vi "Autonomous State Machine Tote.vi"   [LabVIEW 2014]
doc: "This VI is called when autonomous begins, and will automatically be terminated when autonomous ends. You can carry out timed or sensor driven robot movement independently without needing to return to the caller."
uses:
  <vilib>/Rock Robotics/WPI/RobotDrive/WPI_RobotDriveGetSetRefNum.vi
panel:
  # "Be sure to right-click and choose Data Operations>>Make Current Value default if you want to save the array values with the VI"
types:
  T1 = typedef "WPI_MotorControlDeviceRef.ctl" = cluster{"DeviceStatus":errorcluster, "Type":T2, "PWM":cluster{"Controller":T3, "PWM Channel":T4, "DeadBand":T5}, "CAN":cluster{"Device Number":u8, "Control Mode":T6, "Semaphore":T7, "Max Vout":dbl, "TalonSRX Control Mode":T8}, "Invert":bool, "TransformRef":T9, "InvTransformRef":T9}
  T2 = typedef "WPI_MotorControlType.ctl" = enum16{"PWM", "CAN", "CANTalonSRX"}
  T3 = typedef "FPGA_TypedefDigitalModule.ctl" = enum16{"Controller 1"}
  T4 = typedef "FPGA_DIOPWMChannel.ctl" = enum8{"PWM 0", "PWM 1", "PWM 2", "PWM 3", "PWM 4", "PWM 5", "PWM 6", "PWM 7", "PWM 8", "PWM 9", "PWM MXP 0", "PWM MXP 1", "PWM MXP 2", "PWM MXP 3", "PWM MXP 4", "PWM MXP 5", "PWM MXP 6", "PWM MXP 7", "PWM MXP 8", "PWM MXP 9", "Invalid"}
  T5 = typedef "WPI_PWMDeadband.ctl" = cluster{"Name":string, "maxPositivePwm":i32, "minPositivePwm":i32, "centerPwm":i32, "maxNegativePwm":i32, "minNegativePwm":i32, "angularRange":u16}
  T6 = typedef "WPI_CANJaguar_ControlMode.ctl" = enum8{"Percent VBus", "Current", "Speed", "Position", "Voltage"}
  T7 = typedef "Semaphore RefNum" = refnum<k1>
  T8 = typedef "WPI_CANTalonSRX_APIControlMode.ctl" = enum8{"Percent VBus", "Speed", "Position", "Slave", "Unchanged / Invalid"}
  T9 = typedef "WPI_PWMTransform_ConPane.ctl" = refnum<vi>
  T10 = typedef "WPI_RobotDriveDevRef.ctl" = cluster{"DevStatus":errorcluster, "Motors[]":T1[], "Square Inputs":bool, "Max Output":dbl}
  T11 = typedef "WPI_SwitchDevRef.ctl" = cluster{"DevStatus":errorcluster, "DIO Channel":T12, "Controller":T3, "CntIndex":T13, "Normally Closed":bool}
  T12 = typedef "FPGA_DIOChannel.ctl" = enum8{"DIO 0", "DIO 1", "DIO 2", "DIO 3", "DIO 4", "DIO 5", "DIO 6", "DIO 7", "DIO 8", "DIO 9", "DIO MXP 0", "DIO MXP 1", "DIO MXP 2", "DIO MXP 3", "DIO MXP 4", "DIO MXP 5", "DIO MXP 6", "DIO MXP 7", "DIO MXP 8", "DIO MXP 9", "DIO MXP 10", "DIO MXP 11", "DIO MXP 12", "DIO MXP 13", "DIO MXP 14", "DIO MXP 15", "Invalid"}
  T13 = typedef "FPGA_CounterCtrSystemIndex.ctl" = enum8{"Ctr 0", "Ctr 1", "Ctr 2", "Ctr 3", "Ctr 4", "Ctr 5", "Ctr 6", "Ctr 7", "Invalid"}
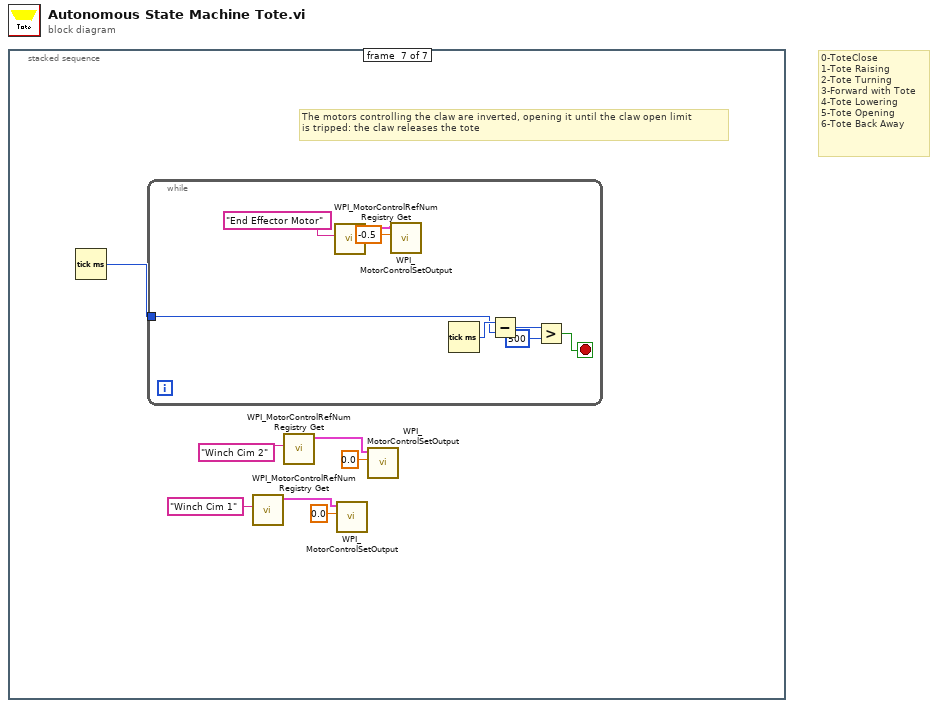
[diagram p0: block diagram]
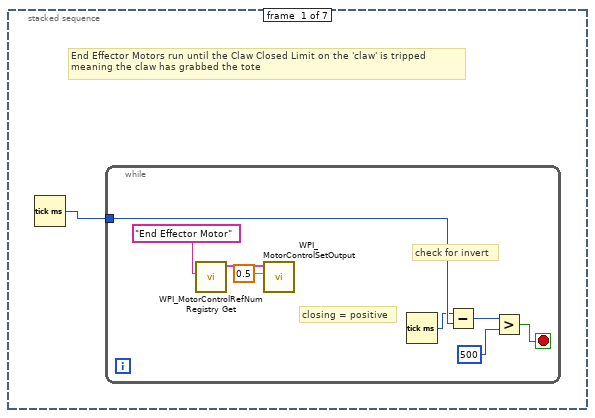
[diagram p2: hidden frame]
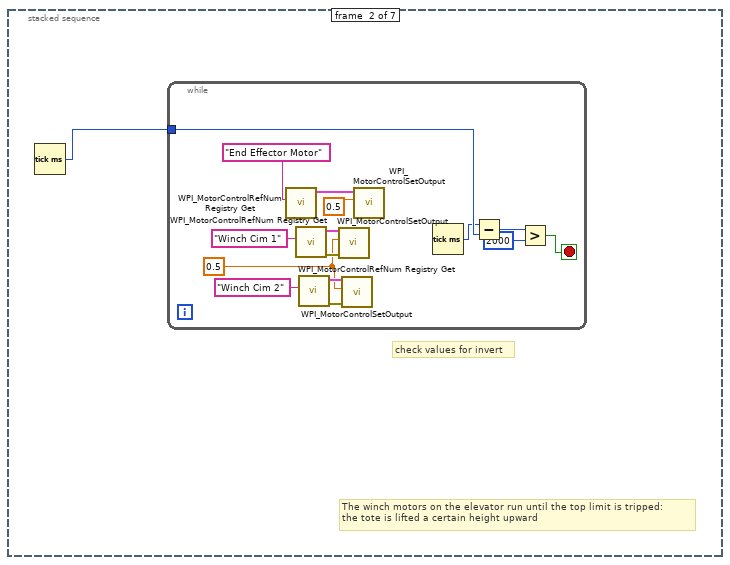
[diagram p3: hidden frame]
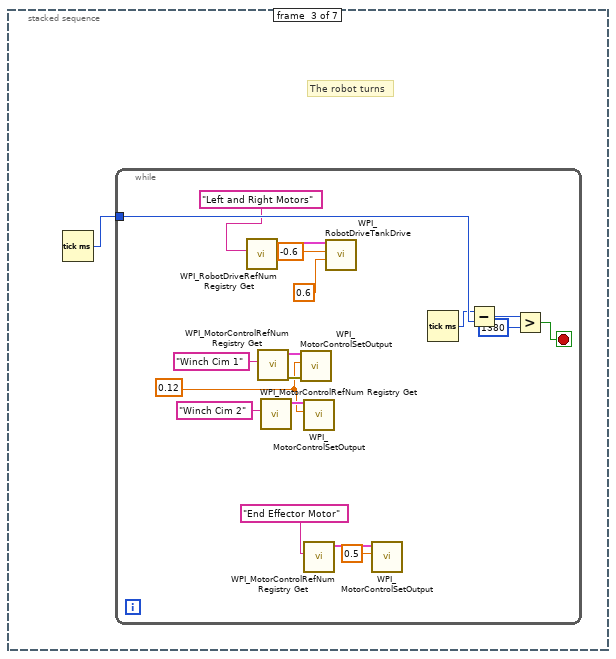
[diagram p4: hidden frame]
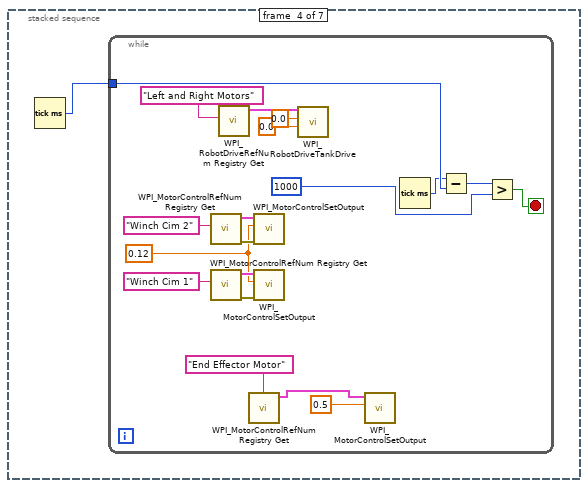
[diagram p5: hidden frame]
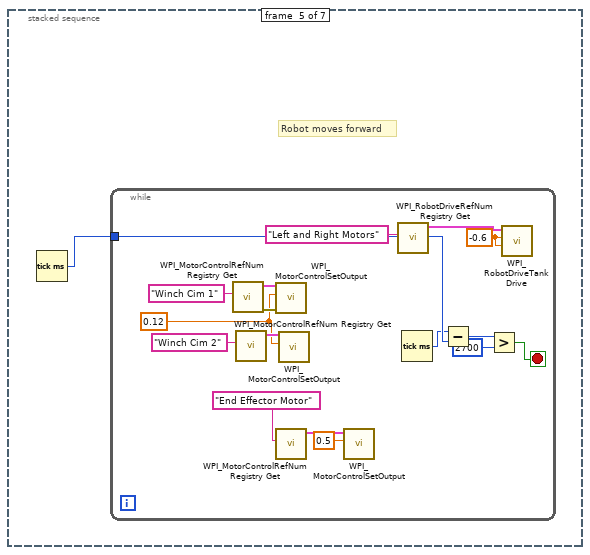
[diagram p6: hidden frame]
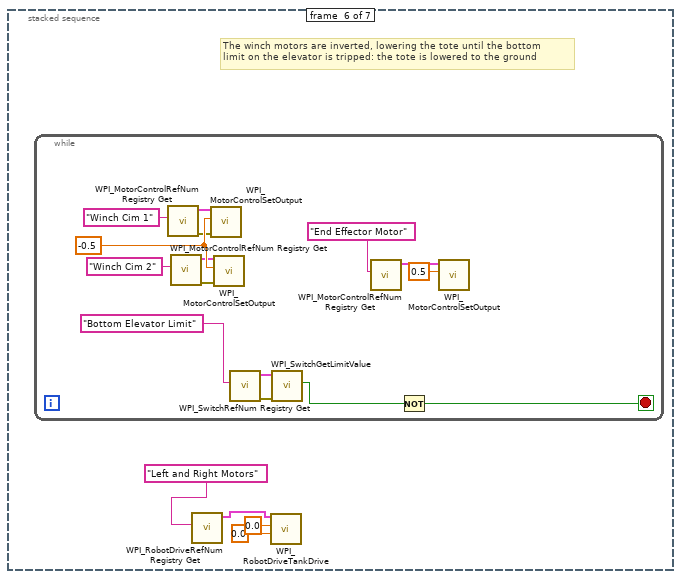
[diagram p7: hidden frame]
diagram:
  # "0-ToteClose\n1-Tote Raising\n2-Tote Turning\n3-Forward with Tote\n4-Tote Lowering\n5-Tote Opening\n6-Tote Back Away"
  n1 = stacked-sequence {
    frame #0 {
      # "End Effector Motors run until the Claw Closed Limit on the 'claw' is tripped\nmeaning the claw has grabbed the tote"
      n2 = Tick Count (ms)() -> (millisecond timer value=w1:u32)
      n3 = while {
        tunnel: w1 -> [w6]
        stop <- w7 stop-if-true
        # "closing = positive"
        # "check for invert"
        n4 = call <vilib>:"WPI_MotorControlRefNum Registry Get.vi"("refnum name"="End Effector Motor") -> ("MotorControlDevRef"=w2:T1)  [unwired: 9 in, 1 out]
        n5 = call <vilib>:"WPI_MotorControlSetOutput.vi"("Output"=0.5, "MotorControlDevRef"=w2) -> ()  [unwired: 7 in, 3 out]
        n6 = Tick Count (ms)() -> (millisecond timer value=w5:u32)
        n7 = Subtract(x=w5, y=w6) -> (x-y=w9:u32)
        n8 = Greater?(x=w9, y=u32 500) -> (0:w7:bool)
      }
    }
    frame #1 {
      # "The winch motors on the elevator run until the top limit is tripped: \nthe tote is lifted a certain height upward"
      # "check values for invert"
      n9 = Tick Count (ms)() -> (millisecond timer value=w10:u32)
      n10 = while {
        tunnel: w10 -> [w22]
        stop <- w23 stop-if-true
        w14 = 0.5
        n11 = call <vilib>:"WPI_MotorControlRefNum Registry Get.vi"("refnum name"="End Effector Motor") -> ("MotorControlDevRef"=w13:T1)  [unwired: 9 in, 1 out]
        n12 = call <vilib>:"WPI_MotorControlRefNum Registry Get.vi"("refnum name"="Winch Cim 1") -> ("error out"=w19:errorcluster, "MotorControlDevRef"=w18:T1)  [unwired: 9 in]
        n13 = call <vilib>:"WPI_MotorControlRefNum Registry Get.vi"("refnum name"="Winch Cim 2") -> ("error out"=w16:errorcluster, "MotorControlDevRef"=w15:T1)  [unwired: 9 in]
        n14 = call <vilib>:"WPI_MotorControlSetOutput.vi"("error in (no error)"=w19, "Output"=w14, "MotorControlDevRef"=w18) -> ()  [unwired: 6 in, 3 out]
        n15 = call <vilib>:"WPI_MotorControlSetOutput.vi"("error in (no error)"=w16, "Output"=w14, "MotorControlDevRef"=w15) -> ()  [unwired: 6 in, 3 out]
        n16 = call <vilib>:"WPI_MotorControlSetOutput.vi"("Output"=0.5, "MotorControlDevRef"=w13) -> ()  [unwired: 7 in, 3 out]
        n17 = Tick Count (ms)() -> (millisecond timer value=w21:u32)
        n18 = Subtract(x=w21, y=w22) -> (x-y=w25:u32)
        n19 = Greater?(x=w25, y=u32 2000) -> (0:w23:bool)
      }
    }
    frame #2 {
      # "The robot turns"
      n20 = Tick Count (ms)() -> (millisecond timer value=w26:u32)
      n21 = while {
        tunnel: w26 -> [w41]
        stop <- w42 stop-if-true
        w31 = 0.12
        n22 = call <vilib>:"WPI_RobotDriveRefNum Registry Get.vi"("refnum name"="Left and Right Motors") -> ("RobotDriveDevRef"=w39:T10)  [unwired: 9 in, 1 out]
        n23 = call <vilib>:"WPI_MotorControlRefNum Registry Get.vi"("refnum name"="Winch Cim 1") -> ("error out"=w34:errorcluster, "MotorControlDevRef"=w30:T1)  [unwired: 9 in]
        n24 = call <vilib>:"WPI_MotorControlRefNum Registry Get.vi"("refnum name"="Winch Cim 2") -> ("MotorControlDevRef"=w32:T1)  [unwired: 9 in, 1 out]
        n25 = call <vilib>:"WPI_MotorControlSetOutput.vi"("error in (no error)"=w34, "Output"=w31, "MotorControlDevRef"=w30) -> ()  [unwired: 6 in, 3 out]
        n26 = call <vilib>:"WPI_MotorControlSetOutput.vi"("Output"=w31, "MotorControlDevRef"=w32) -> ()  [unwired: 7 in, 3 out]
        n27 = call <vilib>:"WPI_MotorControlRefNum Registry Get.vi"("refnum name"="End Effector Motor") -> ("MotorControlDevRef"=w27:T1)  [unwired: 9 in, 1 out]
        n28 = call <vilib>:"WPI_RobotDriveTankDrive.vi"("Right axis value"=0.6, "Left axis value"=-0.6, "RobotDriveDevRef"=w39) -> ()  [unwired: 6 in, 3 out]
        n29 = call <vilib>:"WPI_MotorControlSetOutput.vi"("Output"=0.5, "MotorControlDevRef"=w27) -> ()  [unwired: 7 in, 3 out]
        n30 = Tick Count (ms)() -> (millisecond timer value=w40:u32)
        n31 = Subtract(x=w40, y=w41) -> (x-y=w44:u32)
        n32 = Greater?(x=w44, y=u32 1380) -> (0:w42:bool)
      }
    }
    frame #3 {
      n33 = Tick Count (ms)() -> (millisecond timer value=w45:u32)
      n34 = while {
        tunnel: w45 -> [w62]
        stop <- w63 stop-if-true
        w49 = 0.12
        n35 = call <vilib>:"WPI_MotorControlRefNum Registry Get.vi"("refnum name"="Winch Cim 2") -> ("error out"=w51:errorcluster, "MotorControlDevRef"=w50:T1)  [unwired: 9 in]
        n36 = call <vilib>:"WPI_MotorControlRefNum Registry Get.vi"("refnum name"="Winch Cim 1") -> ("error out"=w54:errorcluster, "MotorControlDevRef"=w53:T1)  [unwired: 9 in]
        n37 = call <vilib>:"WPI_RobotDriveRefNum Registry Get.vi"("refnum name"="Left and Right Motors") -> ("RobotDriveDevRef"=w60:T10)  [unwired: 9 in, 1 out]
        n38 = call <vilib>:"WPI_MotorControlRefNum Registry Get.vi"("refnum name"="End Effector Motor") -> ("MotorControlDevRef"=w46:T1)  [unwired: 9 in, 1 out]
        n39 = call <vilib>:"WPI_MotorControlSetOutput.vi"("error in (no error)"=w51, "Output"=w49, "MotorControlDevRef"=w50) -> ()  [unwired: 6 in, 3 out]
        n40 = call <vilib>:"WPI_MotorControlSetOutput.vi"("error in (no error)"=w54, "Output"=w49, "MotorControlDevRef"=w53) -> ()  [unwired: 6 in, 3 out]
        n41 = call <vilib>:"WPI_RobotDriveTankDrive.vi"("Right axis value"=0.0, "Left axis value"=0.0, "RobotDriveDevRef"=w60) -> ()  [unwired: 6 in, 3 out]
        n42 = call <vilib>:"WPI_MotorControlSetOutput.vi"("Output"=0.5, "MotorControlDevRef"=w46) -> ()  [unwired: 7 in, 3 out]
        n43 = Tick Count (ms)() -> (millisecond timer value=w61:u32)
        n44 = Subtract(x=w61, y=w62) -> (x-y=w64:u32)
        n45 = Greater?(x=w64, y=1000) -> (0:w63:bool)
      }
    }
    frame #4 {
      # "Robot moves forward"
      n46 = Tick Count (ms)() -> (millisecond timer value=w65:u32)
      n47 = while {
        tunnel: w65 -> [w79]
        stop <- w80 stop-if-true
        w70 = 0.12
        w75 = -0.6 ("Left axis value")
        n48 = call <vilib>:"WPI_MotorControlRefNum Registry Get.vi"("refnum name"="Winch Cim 1") -> ("error out"=w73:errorcluster, "MotorControlDevRef"=w69:T1)  [unwired: 9 in]
        n49 = call <vilib>:"WPI_MotorControlRefNum Registry Get.vi"("refnum name"="Winch Cim 2") -> ("MotorControlDevRef"=w71:T1)  [unwired: 9 in, 1 out]
        n50 = call <vilib>:"WPI_MotorControlSetOutput.vi"("error in (no error)"=w73, "Output"=w70, "MotorControlDevRef"=w69) -> ()  [unwired: 6 in, 3 out]
        n51 = call <vilib>:"WPI_MotorControlRefNum Registry Get.vi"("refnum name"="End Effector Motor") -> ("MotorControlDevRef"=w66:T1)  [unwired: 9 in, 1 out]
        n52 = call <vilib>:"WPI_MotorControlSetOutput.vi"("Output"=w70, "MotorControlDevRef"=w71) -> ()  [unwired: 7 in, 3 out]
        n53 = call <vilib>:"WPI_MotorControlSetOutput.vi"("Output"=0.5, "MotorControlDevRef"=w66) -> ()  [unwired: 7 in, 3 out]
        n54 = call <vilib>:"WPI_RobotDriveRefNum Registry Get.vi"("refnum name"="Left and Right Motors") -> ("RobotDriveDevRef"=w77:T10)  [unwired: 9 in, 1 out]
        n55 = Tick Count (ms)() -> (millisecond timer value=w78:u32)
        n56 = Subtract(x=w78, y=w79) -> (x-y=w82:u32)
        n57 = Greater?(x=w82, y=u32 2700) -> (0:w80:bool)
        n58 = call <vilib>:"WPI_RobotDriveTankDrive.vi"("Right axis value"=w75, "Left axis value"=w75, "RobotDriveDevRef"=w77) -> ()  [unwired: 6 in, 3 out]
      }
    }
    frame #5 {
      # "The winch motors are inverted, lowering the tote until the bottom \nlimit on the elevator is tripped: the tote is lowered to the ground"
      n59 = while {
        stop <- w90 stop-if-true
        w101 = -0.5
        n60 = call <vilib>:"WPI_MotorControlRefNum Registry Get.vi"("refnum name"="Winch Cim 1") -> ("error out"=w96:errorcluster, "MotorControlDevRef"=w97:T1)  [unwired: 9 in]
        n61 = call <vilib>:"WPI_MotorControlRefNum Registry Get.vi"("refnum name"="Winch Cim 2") -> ("error out"=w99:errorcluster, "MotorControlDevRef"=w100:T1)  [unwired: 9 in]
        n62 = call <vilib>:"WPI_MotorControlSetOutput.vi"("error in (no error)"=w96, "Output"=w101, "MotorControlDevRef"=w97) -> ()  [unwired: 6 in, 3 out]
        n63 = call <vilib>:"WPI_MotorControlSetOutput.vi"("error in (no error)"=w99, "Output"=w101, "MotorControlDevRef"=w100) -> ()  [unwired: 6 in, 3 out]
        n64 = call <vilib>:"WPI_SwitchRefNum Registry Get.vi"("refnum name"="Bottom Elevator Limit") -> ("error out"=w94:errorcluster, "SwitchDevRef"=w93:T11)  [unwired: 9 in]
        n65 = call <vilib>:"WPI_SwitchGetLimitValue.vi"("error in (no error)"=w94, "SwitchDevRef"=w93) -> ("Switch Pressed"=w91:bool)  [unwired: 7 in, 2 out]
        n66 = call <vilib>:"WPI_MotorControlRefNum Registry Get.vi"("refnum name"="End Effector Motor") -> ("MotorControlDevRef"=w87:T1)  [unwired: 9 in, 1 out]
        n67 = Not(x=w91) -> (.not. x?=w90:bool)
        n68 = call <vilib>:"WPI_MotorControlSetOutput.vi"("Output"=0.5, "MotorControlDevRef"=w87) -> ()  [unwired: 7 in, 3 out]
      }
      n69 = call <vilib>:"WPI_RobotDriveRefNum Registry Get.vi"("refnum name"="Left and Right Motors") -> ("RobotDriveDevRef"=w86:T10)  [unwired: 9 in, 1 out]
      n70 = call <vilib>:"WPI_RobotDriveTankDrive.vi"("Right axis value"=0.0, "Left axis value"=0.0, "RobotDriveDevRef"=w86) -> ()  [unwired: 6 in, 3 out]
    }
    frame #6 {
      # "The motors controlling the claw are inverted, opening it until the claw open limit\nis tripped: the claw releases the tote"
      n71 = Tick Count (ms)() -> (millisecond timer value=w108:u32)
      n72 = while {
        tunnel: w108 -> [w109]
        stop <- w114 stop-if-true
        n73 = call <vilib>:"WPI_MotorControlRefNum Registry Get.vi"("refnum name"="End Effector Motor") -> ("MotorControlDevRef"=w111:T1)  [unwired: 9 in, 1 out]
        n74 = call <vilib>:"WPI_MotorControlSetOutput.vi"("Output"=-0.5, "MotorControlDevRef"=w111) -> ()  [unwired: 7 in, 3 out]
        n75 = Tick Count (ms)() -> (millisecond timer value=w113:u32)
        n76 = Subtract(x=w113, y=w109) -> (x-y=w116:u32)
        n77 = Greater?(x=w116, y=u32 500) -> (0:w114:bool)
      }
      n78 = call <vilib>:"WPI_MotorControlRefNum Registry Get.vi"("refnum name"="Winch Cim 1") -> ("MotorControlDevRef"=w103:T1)  [unwired: 9 in, 1 out]
      n79 = call <vilib>:"WPI_MotorControlRefNum Registry Get.vi"("refnum name"="Winch Cim 2") -> ("MotorControlDevRef"=w106:T1)  [unwired: 9 in, 1 out]
      n80 = call <vilib>:"WPI_MotorControlSetOutput.vi"("Output"=0.0, "MotorControlDevRef"=w103) -> ()  [unwired: 7 in, 3 out]
      n81 = call <vilib>:"WPI_MotorControlSetOutput.vi"("Output"=0.0, "MotorControlDevRef"=w106) -> ()  [unwired: 7 in, 3 out]
    }
  }
